vi "failsound.vi"(8 "error in":errorcluster) -> (0 "error out":errorcluster)   [LabVIEW 2024]
uses:
  <vilib>/sound2/lvsound2.llb/Sampling Mode.ctl
  <vilib>/sound2/lvsound2.llb/Sound File Info (path).vi
  <vilib>/sound2/lvsound2.llb/Sound File Read Open.vi
  <vilib>/sound2/lvsound2.llb/Sound File Read (DBL).vi
  <vilib>/sound2/lvsound2.llb/Sound Output Write (DBL).vi
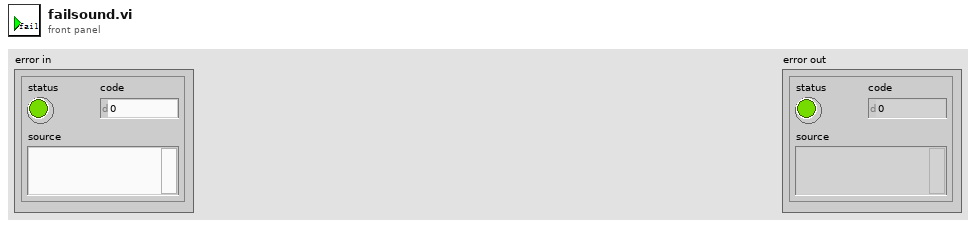
[diagram p1: front panel]
types:
  T1 = typedef "Sampling Mode.ctl" = i32
  T2 = typedef "Sound Data Format.ctl" = cluster{"sample rate (S/s)":dbl, "number of channels":i32, "bits per sample":i32}
  T3 = typedef "Sound File Refnum.ctl" = refnum<file>
  T4 = typedef "Sound Output Task ID.ctl" = u32
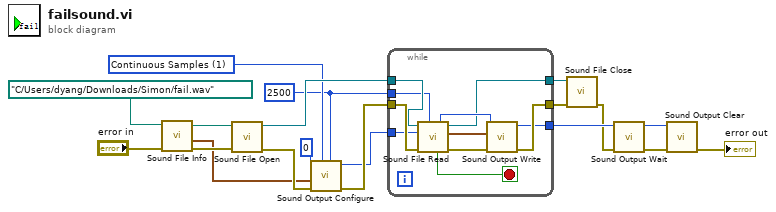
[diagram p0: block diagram]
diagram:
  w3 = 2500 ("number of samples/ch")
  w4 = T1 1 items=["Finite Samples", "Continuous Samples"] ("sample mode")
  n1 = call-poly <vilib>:"Sound File Info.vi"("error in (no error)"="error in", "path"=path "C:/Users/dyang/Downloads/Simon/fail.wav") -> ("error out"=w17:errorcluster, "sound format"=w15:T2, "path out"=w18:path)  [unwired: 6 in, 1 out]
  n2 = call-poly <vilib>:"Sound File Open.vi"("error in (no error)"=w17, "path"=w18) -> ("error out"=w16:errorcluster, "sound file refnum"=w13:T3)  [unwired: 8 in]
  n3 = call <vilib>:"Sound Output Configure.vi"("number of samples/ch"=w3, "sample mode"=w4, "error in (no error)"=w16, "sound format"=w15, "device ID"=u32 0) -> ("error out"=w12:errorcluster, "task ID"=w11:T4)  [unwired: 5 in]
  n4 = while {
    tunnel: w3 -> [w22]
    tunnel: w13 -> [w29]
    tunnel: [w25] -> w10
    tunnel: w12 -> [w28]
    tunnel: [w24] -> w9
    tunnel: w11 -> [w26]
    tunnel: [w23] -> w8
    stop <- w20 stop-if-true
    n5 = call-poly <vilib>:"Sound File Read.vi"("number of samples/ch (-1: all)"=w22, "error in (no error)"=w28, "sound file refnum"=w29) -> ("error out"=w27:errorcluster, "data"=w21:waveform(dbl)[], "sound file refnum out"=w25:T3, "end of file?"=w20:bool)  [unwired: 4 in, 1 out]
    n6 = call-poly <vilib>:"Sound Output Write.vi"("error in (no error)"=w27, "data"=w21, "task ID"=w26) -> ("error out"=w24:errorcluster, "task ID out"=w23:T4)  [unwired: 7 in]
  }
  n7 = call <vilib>:"Sound File Close.vi"("error in (no error)"=w9, "sound file refnum"=w10) -> ("error out"=w7:errorcluster)  [unwired: 9 in]
  n8 = call <vilib>:"Sound Output Wait.vi"("error in (no error)"=w7, "task ID"=w8) -> ("error out"=w6:errorcluster, "task ID out"=w5:T4)  [unwired: 8 in]
  n9 = call <vilib>:"Sound Output Clear.vi"("error in (no error)"=w6, "task ID"=w5) -> ("error out"=→"error out":errorcluster)  [unwired: 9 in]
